vi "Connect_AMI.vi"() -> ()   [LabVIEW 2016]
uses:
  Instrument_Setup.vi
panel:
  in  "error in":T1
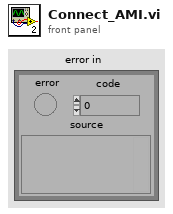
[diagram p1: front panel]
types:
  T1 = cluster{"error":bool, "code":i32, "source":string}
  T2 = cluster{"GPIB address":i16, "GPIB bus":i16, "connection ID":refnum<k5>, "IP":string, "Active Comm Interface":u16, "Serial Port":refnum<visa-resource-name>, "Programmer Type":u16}
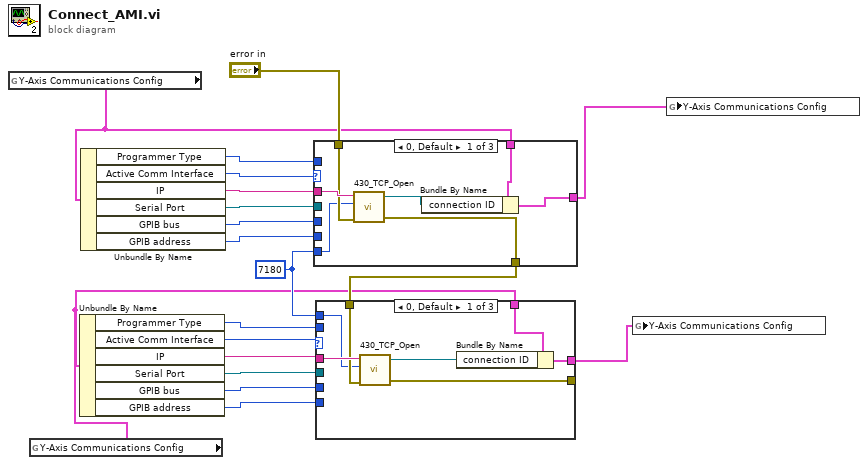
[diagram p0: block diagram]
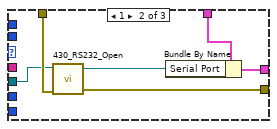
[diagram p2: hidden frame]
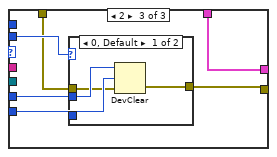
[diagram p3: hidden frame]
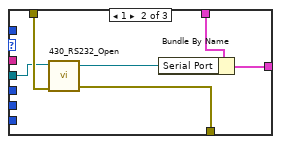
[diagram p5: hidden frame]
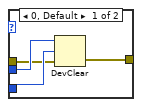
[diagram p7: hidden frame]
diagram:
  w19 = 7180 ("TCP Port")
  n1 = global read "Instrument_Setup.vi" "Y-Axis Communications Config"() -> (w4:T2)
  n2 = global read "Instrument_Setup.vi" "Y-Axis Communications Config"() -> (w3:T2)
  n3 = Unbundle By Name(w3) -> ("Programmer Type"=w12:u16, "Active Comm Interface"=w18:u16, "IP"=w15:string, "Serial Port"=w14:refnum<visa-resource-name>, "GPIB bus"=w11:i16, "GPIB address"=w10:i16)
  n4 = Unbundle By Name(w4) -> ("Programmer Type"=w6:u16, "Active Comm Interface"=w17:u16, "IP"=w16:string, "Serial Port"=w13:refnum<visa-resource-name>, "GPIB bus"=w7:i16, "GPIB address"=w8:i16)
  n5 = case shown="0, Default" w17 {
    tunnel: w16 -> [w26 _ _]
    tunnel: "error in" -> [w25 w32 w34]
    tunnel: w4 -> [w24 w27 w38]
    tunnel: [w22 w30 w38] -> w2
    tunnel: [w21 w31 w33] -> w9
    tunnel: w19 -> [w20 _ _]
    tunnel: w13 -> [_ w28 _]
    tunnel: w8 -> [_ _ w37]
    tunnel: w7 -> [_ _ w36]
    tunnel: w6 -> [_ _ w35]
    frame 0, Default {
      n6 = call "430_TCP_Open.vi"("IP Address"=w26, "TCP Port"=w20, "error in (no error)"=w25) -> ("connection ID"=w23:refnum<k5>, "error out"=w21:errorcluster)  [unwired: 3 in, 1 out]
      n7 = Bundle By Name(cluster=w24, "connection ID"=w23) -> (w22:T2)
    }
    frame 1 {
      n8 = call "430_RS232_Open.vi"("VISA resource name"=w28, "error in (no error)"=w32) -> ("VISA resource name out"=w29:refnum<visa-resource-name>, "error out"=w31:errorcluster)  [unwired: 5 in]
      n9 = Bundle By Name(cluster=w27, "Serial Port"=w29) -> (w30:T2)
    }
    frame 2 {
      n10 = case shown="1" w35 {
        tunnel: w36 -> [w42 _]
        tunnel: w37 -> [w41 _]
        tunnel: w34 -> [w40 w43]
        tunnel: [w39 w43] -> w33
        frame 0, Default {
          n11 = DevClear(2:w40, 3:w41, 4:w42) -> (0:w39:errorcluster)  [unwired: 1 out]
        }
        frame 1 {
        }
      }
    }
  }
  n12 = case shown="0, Default" w18 {
    tunnel: w15 -> [w50 _ _]
    tunnel: w9 -> [w49 w56 w58]
    tunnel: [w48 w55 w57] -> _
    tunnel: w3 -> [w47 w53 w62]
    tunnel: [w45 w54 w62] -> w1
    tunnel: w19 -> [w44 _ _]
    tunnel: w14 -> [_ w51 _]
    tunnel: w12 -> [_ _ w61]
    tunnel: w11 -> [_ _ w60]
    tunnel: w10 -> [_ _ w59]
    frame 0, Default {
      n13 = call "430_TCP_Open.vi"("IP Address"=w50, "TCP Port"=w44, "error in (no error)"=w49) -> ("connection ID"=w46:refnum<k5>, "error out"=w48:errorcluster)  [unwired: 3 in, 1 out]
      n14 = Bundle By Name(cluster=w47, "connection ID"=w46) -> (w45:T2)
    }
    frame 1 {
      n15 = call "430_RS232_Open.vi"("VISA resource name"=w51, "error in (no error)"=w56) -> ("VISA resource name out"=w52:refnum<visa-resource-name>, "error out"=w55:errorcluster)  [unwired: 5 in]
      n16 = Bundle By Name(cluster=w53, "Serial Port"=w52) -> (w54:T2)
    }
    frame 2 {
      n17 = case shown="0, Default" w61 {
        tunnel: w60 -> [w66 _]
        tunnel: w59 -> [w65 _]
        tunnel: w58 -> [w64 w67]
        tunnel: [w63 w67] -> w57
        frame 0, Default {
          n18 = DevClear(2:w64, 3:w65, 4:w66) -> (0:w63:errorcluster)  [unwired: 1 out]
        }
        frame 1 {
        }
      }
    }
  }
  n19 = global write "Instrument_Setup.vi" "Y-Axis Communications Config"(w1) -> ()
  n20 = global write "Instrument_Setup.vi" "Y-Axis Communications Config"(w2) -> ()
